vi "Tester.vi"() -> ()   [LabVIEW 2015, in "Song Queue.xctl"]
uses:
  file/MusicElement/Song/Song Duration.ctl
  Song Queue.xctl
  builds/xctls/Song Queue/Song Queue.lvlibp/app/controls/Queue Song Display.ctl
  builds/xctls/Song Queue/Song Queue.lvlibp/file/classes/Song/Song Duration.ctl
  builds/xctls/Song Queue/Song Queue.lvlibp/app/controls/Dequeue Control.ctl
  builds/xctls/Song Queue/Song Queue.lvlibp
  builds/xctls/Song Queue/Song Queue.lvlibp/file/classes/Song/Song.lvclass
  file/MusicElement/Song/Song.lvclass
panel:
  in  "Song Queue":T1[](xcontrol)
  out "Duration (s)":T2 format="%<%M:%S>T"
  in  "Change":bool=TRUE
  in  "Number Of Songs":i32=20
  in  "stop":bool
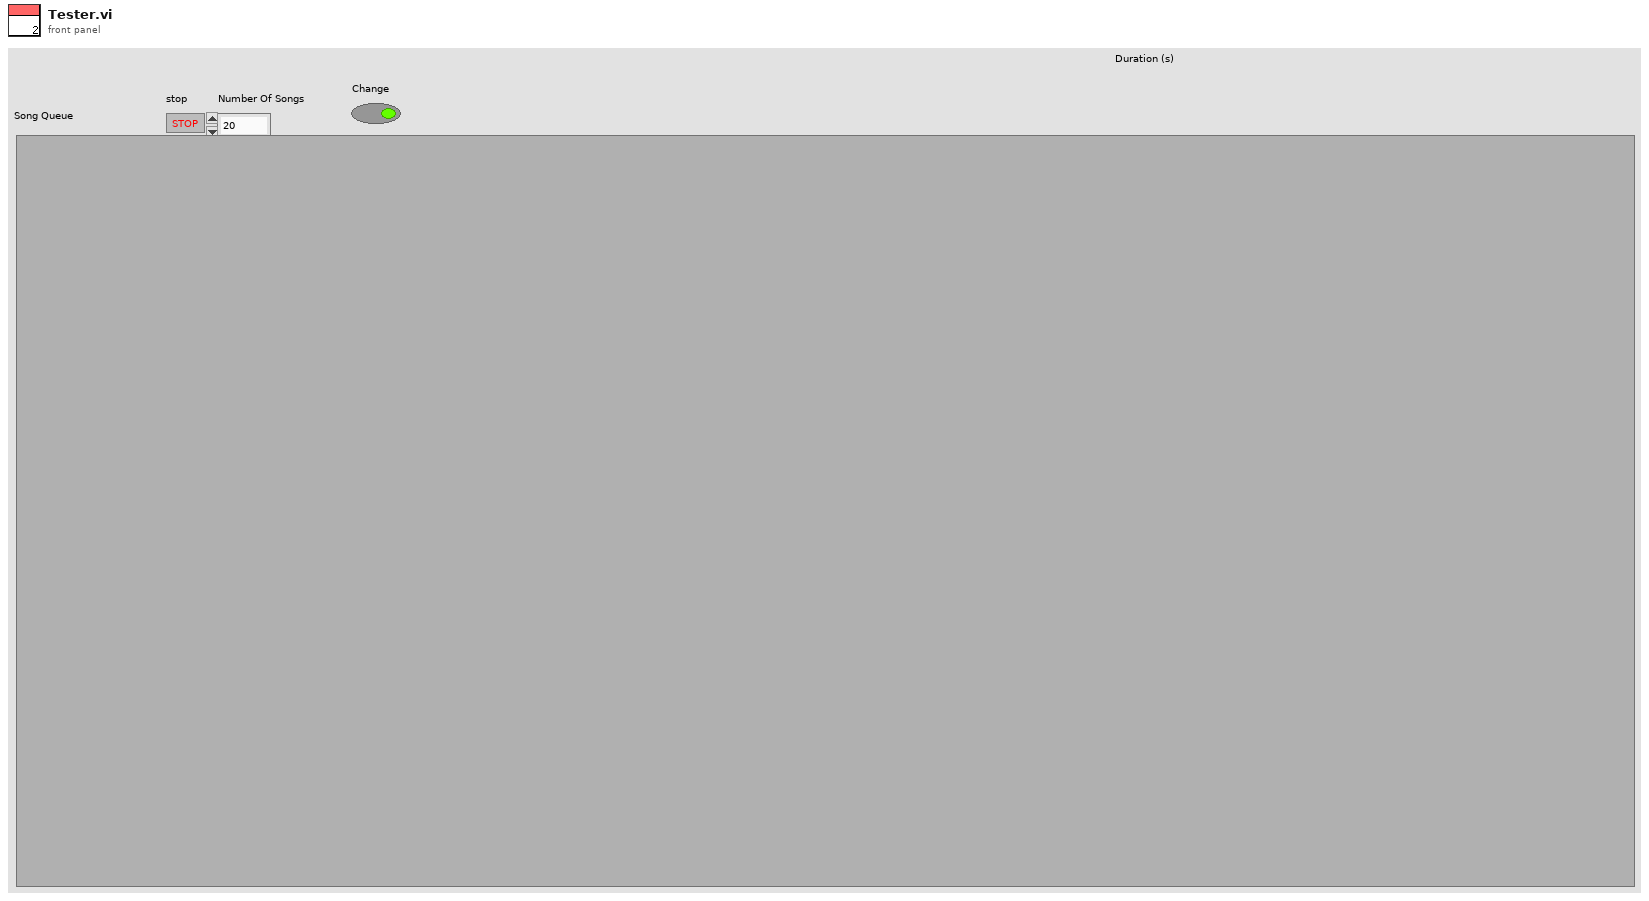
[diagram p1: front panel]
types:
  T1 = typedef "Queue Song Display.ctl" = cluster{"Song Name":string, "Artist":string, "Album":string, "Duration (s)":T2, "UID":string, "Dequeue":T3}
  T2 = typedef "Song.lvclass/Song Duration.ctl" = timestamp
  T3 = typedef "Dequeue Control.ctl" = bool
  T4 = typedef "Song Queue.lvlibp/Queue Song Display.ctl" = cluster{"Song Name":string, "Artist":string, "Album":string, "Duration (s)":T5, "UID":string, "Dequeue":T6}
  T5 = typedef "Song Queue.lvlibp/Song.lvclass/Song Duration.ctl" = timestamp
  T6 = typedef "Song Queue.lvlibp/Dequeue Control.ctl" = bool
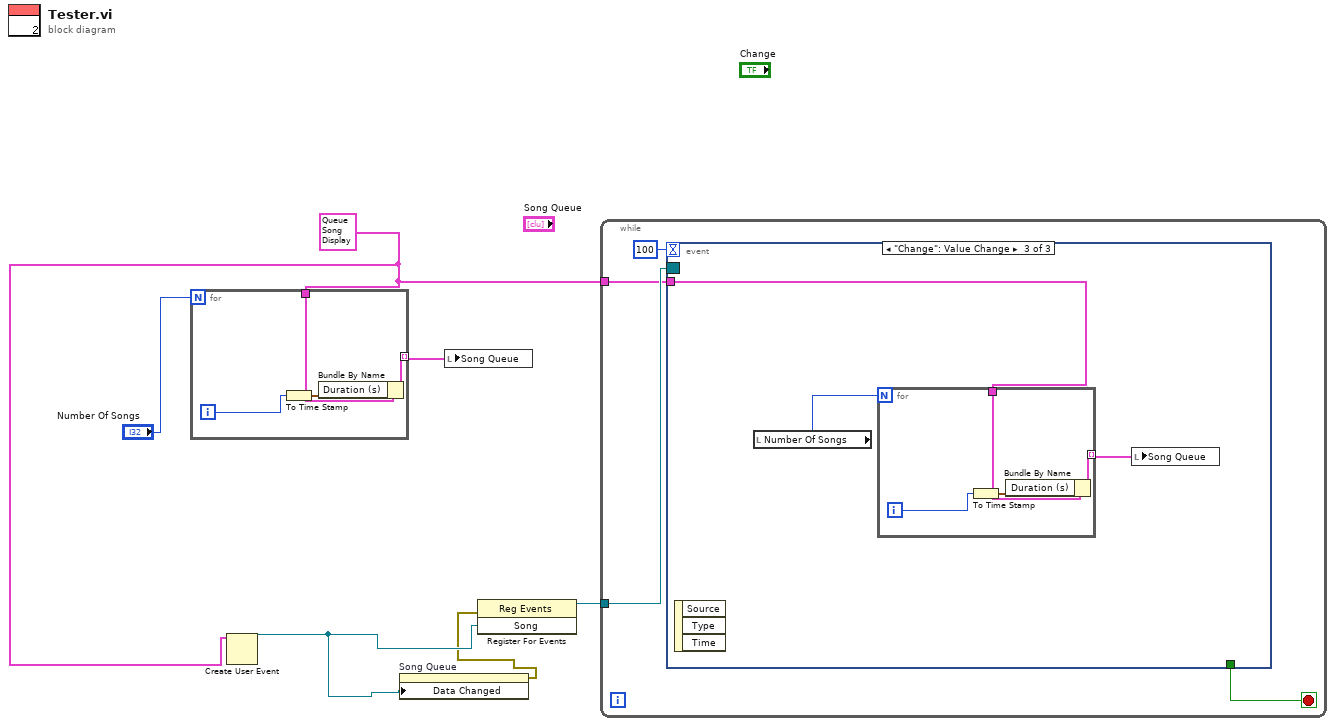
[diagram p0: block diagram]
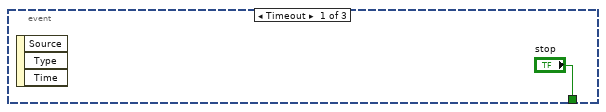
[diagram p2: hidden frame]
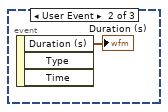
[diagram p3: hidden frame]
diagram:
  w3 = T4 {"Song Name"="", "Artist"="", "Album"="", "Duration (s)"=timestamp(0 s since 1904-01-01), "UID"="", "Dequeue"=FALSE} ("Song")
  n1 = for {
    N: "Number Of Songs" -> [_]
    tunnel: [w10] -> w4 mode=indexing
    tunnel: w3 -> [w7]
    i -> [w9]
    n2 = To Time Stamp(1:w9) -> (0:w8:timestamp)
    n3 = Bundle By Name(cluster=w7, "Duration (s)"=w8) -> (w10:T4)
  }
  n4 = Create User Event(user event datatype=w3) -> (user event=w2:refnum<user-event>)  [unwired: 1 in, 1 out]
  n5 = property on="Song Queue" class="Song Queue (strict)"("Data Changed"=w2) -> (error out=w1:errorcluster)  [unwired: 2 in, 1 out]
  n6 = local write "Song Queue"(w4) -> ()
  n7 = register-events(error in=w1, w2) -> (reference out=w5:refnum<event-registration>)  [unwired: 1 in, 1 out]
  n8 = while {
    tunnel: w5 -> [w12]
    tunnel: w3 -> [w11]
    stop <- w13 stop-if-true
    n9 = event shown="[2] \"Change\": Value Change" {
      selector: w12 -> [_ _ _]
      dyn-events: _ -> [_ _ _]
      timeout: 100 -> [_ _ _]
      tunnel: ["stop" _ _] -> w13
      tunnel: w11 -> [_ _ w18]
      event Timeout {
        n10 = event-data() -> ()  [unwired: 1 in, 3 out]
      }
      event User Event {
        n11 = event-data() -> ("Duration (s)"=→"Duration (s)":T5)  [unwired: 1 in, 2 out]
      }
      event "Change": Value Change {
        n12 = event-data() -> ()  [unwired: 1 in, 3 out]
        n13 = local read "Number Of Songs"() -> (w17:i32)
        n14 = for {
          N: w17 -> [_]
          tunnel: [w23] -> w19 mode=indexing
          tunnel: w18 -> [w20]
          i -> [w22]
          n15 = To Time Stamp(1:w22) -> (0:w21:timestamp)
          n16 = Bundle By Name(cluster=w20, "Duration (s)"=w21) -> (w23:T4)
        }
        n17 = local write "Song Queue"(w19) -> ()
      }
    }
  }
